vi "Mandelbrot_generator.vi"() -> ()   [LabVIEW 2015]
panel:
  out "x-y":dbl
  out "Waveform Chart":dbl(graph)
  out "Data Read":i32
  out "VARIANT IN CASE OF ERROR":variant
  out "Errors":i32
  in  "Reset Picture":bool
  out "Throughput":dbl(graph)
  in  "stop":bool
  out "XY Graph":cluster{"X":dbl, "Y":dbl}[](graph)
  out "error out 2":errorcluster
  out "Number of  Tuples":i32
  in  "Numeric":i32
  in  "Ring":u16(ring) items=["Rworker.vi", ""]
  in  "Async ?":bool
  in  "machine name (\"\":  open local reference)":string
  in  "Cicli":i32=200
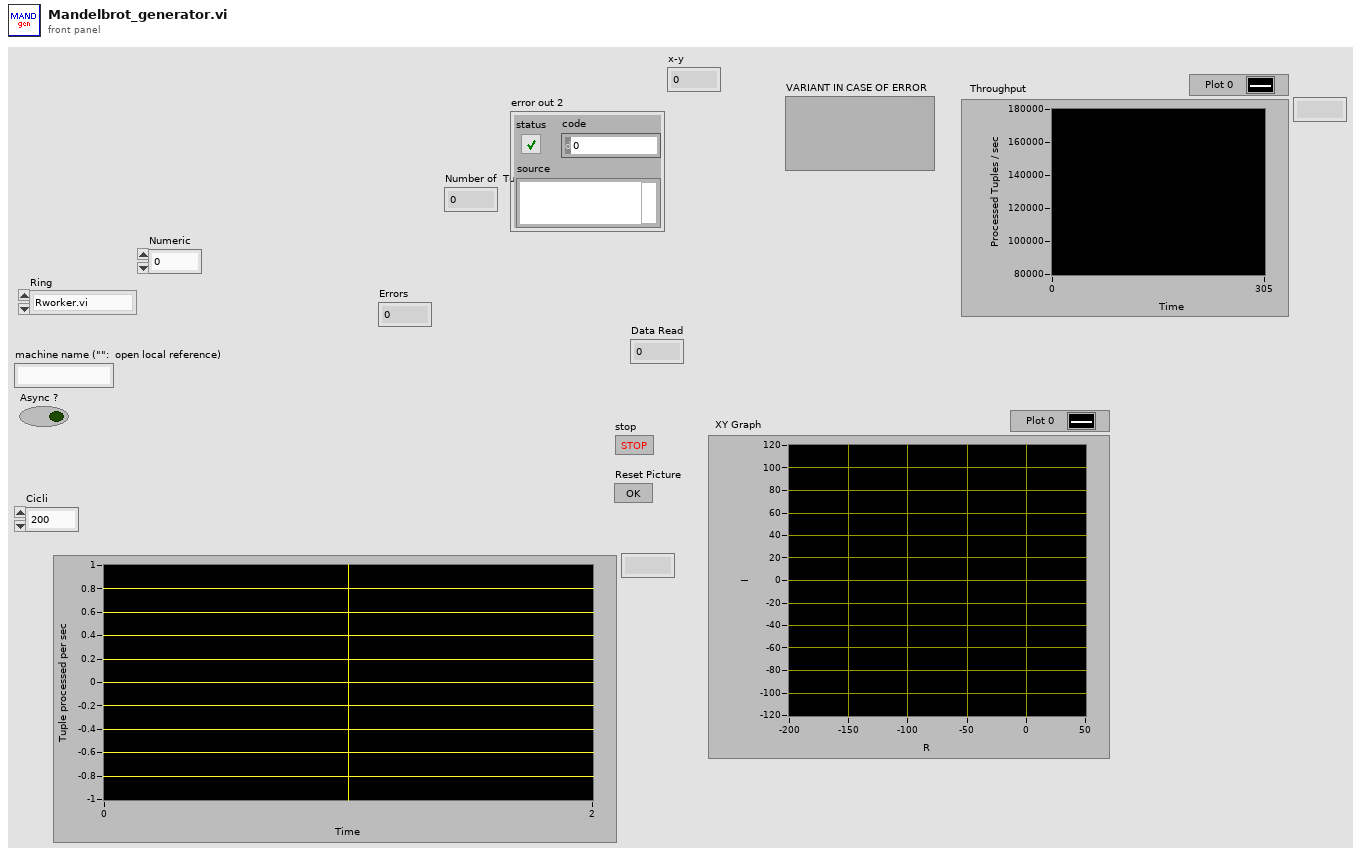
[diagram p1: front panel]
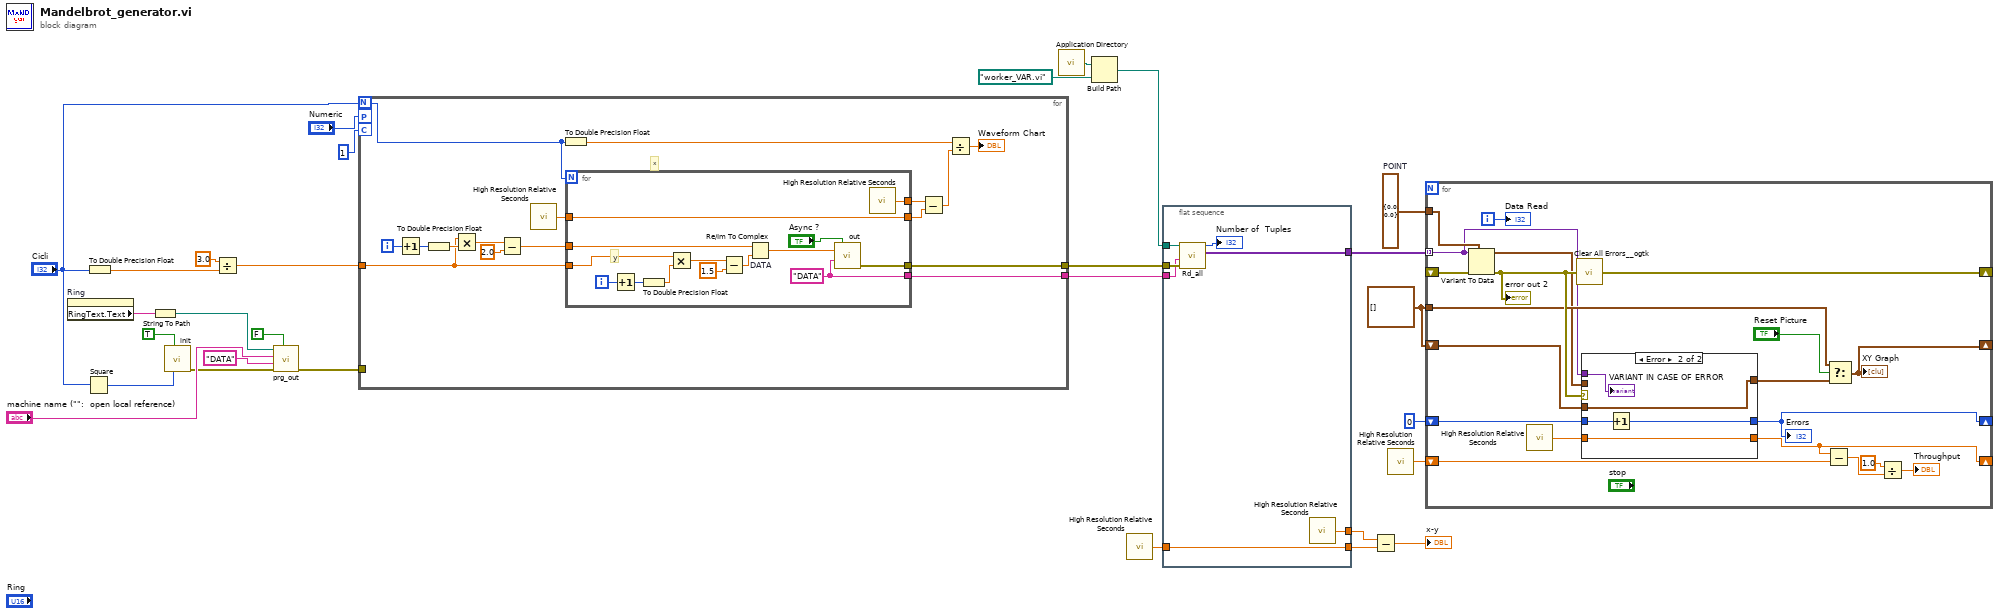
[diagram p0: block diagram]
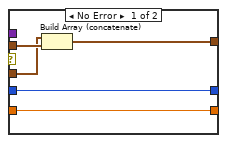
[diagram p2: hidden frame]
diagram:
  w7 = cluster{"X":dbl, "Y":dbl}[] []
  w9 = cluster{"X":dbl, "Y":dbl} {"X"=0.0, "Y"=0.0}  # POINT
  n1 = property on="Ring" class="Ring (strict)"() -> ("RingText.Text"=w17:string)  [unwired: 2 in, 2 out]
  n2 = Square(x="Cicli") -> (x^2=w18:i32)
  n3 = To Double Precision Float(number="Cicli") -> (double precision float=w24:dbl)
  n4 = String To Path(string=w17) -> (path=w23:path)
  n5 = call "init.vi"("Space size"=w18, "Cleaneup"=TRUE ("Cleneup")) -> ("error out"=w20:errorcluster)  [unwired: 9 in]
  n6 = Divide(x=3.0, y=w24) -> (x/y=w28:dbl)
  n7 = call "prg_out.vi"("Reset to default"=FALSE, "error in (no error)"=w20, "Name"="DATA" ("String"), "machine name (\"\":  open local reference)"="machine name (\"\":  open local reference)", "vi path"=w23) -> ("error out"=w26:errorcluster)  [unwired: 6 in]
  n8 = for {
    N: "Cicli" -> [w35]
    tunnel: w28 -> [w44]
    tunnel: w26 -> [_]
    workers-P: "Numeric" -> [_]
    chunk-C: 1 -> [_]
    tunnel: [w32] -> w14
    tunnel: [w31] -> w10
    i -> [w42]
    # "x"
    n9 = Increment(x=w42) -> (x+1=w39:i32)
    n10 = To Double Precision Float(number=w39) -> (double precision float=w45:dbl)
    n11 = Multiply(x=w44, y=w45) -> (x*y=w40:dbl)
    n12 = Subtract(x=w40, y=2.0) -> (x-y=w43:dbl)
    n13 = call <vilib>:"High Resolution Relative Seconds.vi"() -> ("relative seconds"=w38:dbl)
    n14 = To Double Precision Float(number=w35) -> (double precision float=w34:dbl)
    n15 = for {
      N: w35 -> [_]
      tunnel: w44 -> [w58]
      tunnel: w43 -> [w55]
      tunnel: [w50] -> w37
      tunnel: [w49] -> w36
      tunnel: w38 -> [w49]
      tunnel: [w47] -> w32
      tunnel: [w46] -> w31
      i -> [w53]
      w46 = "DATA" ("Name out")
      # "y"
      n16 = Increment(x=w53) -> (x+1=w52:i32)
      n17 = To Double Precision Float(number=w52) -> (double precision float=w59:dbl)
      n18 = Multiply(x=w58, y=w59) -> (x*y=w57:dbl)
      n19 = Subtract(x=w57, y=1.5) -> (x-y=w54:dbl)
      n20 = Re/Im To Complex "DATA"(1:w54, 2:w55) -> (0:w51:cdb)
      n21 = call "out.vi"("Async ?"="Async ?", "IN VARIANT"=w51, "Name in"=w46) -> ("error out"=w47:errorcluster)  [unwired: 11 in, 1 out]
      n22 = call <vilib>:"High Resolution Relative Seconds.vi"() -> ("relative seconds"=w50:dbl)
    }
    n23 = Subtract(x=w37, y=w36) -> (x-y=w33:dbl)
    n24 = Divide(x=w34, y=w33) -> (x/y=→"Waveform Chart":dbl)
  }
  n25 = call <vilib>:"Application Directory.vi"() -> ("Application Directory"=w13:path)
  n26 = Build Path(base path=w13, name or relative path=path "worker_VAR.vi" ("vi path")) -> (appended path=w11:path)
  n27 = call <vilib>:"High Resolution Relative Seconds.vi"() -> ("relative seconds"=w4:dbl)
  n28 = flat-sequence {
    tunnel: w14 -> [w66]
    tunnel: w11 -> [w65]
    tunnel: w10 -> [w63]
    tunnel: [w62] -> w5
    tunnel: w4 -> [w60]
    tunnel: [w61] -> w3
    tunnel: [w60] -> w2
    frame #0 {
      n29 = call "Rd_all.vi"("error in (no error)"=w66, "Name in"=w63, "Vi path"=w65) -> ("Rd_all Array"=w62:variant[], "Number of  Tuples"=→"Number of  Tuples":i32)  [unwired: 6 in, 1 out]
      n30 = call <vilib>:"High Resolution Relative Seconds.vi"() -> ("relative seconds"=w61:dbl)
    }
  }
  n31 = Subtract(x=w3, y=w2) -> (x-y=→"x-y":dbl)
  n32 = call <vilib>:"High Resolution Relative Seconds.vi"() -> ("relative seconds"=w6:dbl)
  n33 = for {
    tunnel: w9 -> [w85]
    shift-right: [w72] -> _
    shift-left: w7 -> [w70]
    shift-right: [w84] -> _
    shift-left: _ -> [w67]
    shift-right: [w81] -> _
    shift-left: 0 -> [w82]
    tunnel: w7 -> [w80]
    shift-right: [w77] -> _
    shift-left: w6 -> [w78]
    tunnel: w5 -> [w68] mode=indexing
    i -> [w86]
    n34 = Variant To Data(error in=w67, type=w85, Variant=w68) -> (data=w71:cluster{"X":dbl, "Y":dbl}, error out=w83:errorcluster)
    "error out 2" <- w83
    n35 = call <vilib>:"High Resolution Relative Seconds.vi"() -> ("relative seconds"=w73:dbl)
    n36 = call <userlib>:"Clear All Errors__ogtk.vi"("Error In"=w83) -> ("Error Out"=w84:errorcluster)  [unwired: 3 in]
    n37 = case shown="Error" w83 {
      tunnel: w82 -> [w91 w96]
      tunnel: [w91 w95] -> w81
      tunnel: w68 -> [_ w94]
      tunnel: [w90 w93] -> w77
      tunnel: w73 -> [w90 w93]
      tunnel: w71 -> [w89 _]
      tunnel: w70 -> [w88 w92]
      tunnel: [w87 w92] -> w69
      frame No Error {
        n38 = Build Array (concatenate)(w88, w89) -> (w87:cluster{"X":dbl, "Y":dbl}[])
      }
      frame Error {
        n39 = Increment(x=w96) -> (x+1=w95:i32)
        "VARIANT IN CASE OF ERROR" <- w94
      }
    }
    "Errors" <- w81
    n40 = Subtract(x=w77, y=w78) -> (x-y=w75:dbl)
    n41 = Select(t=w80, s="Reset Picture", f=w69) -> (s? t:f=w72:cluster{"X":dbl, "Y":dbl}[])
    "XY Graph" <- w72
    n42 = Divide(x=1.0, y=w75) -> (x/y=→"Throughput":dbl)
    "Data Read" <- w86
  }
